vi "Get Provided Interface and Service Class.vi"(8 "error in":errorcluster, 11 "instrument in":refnum<class "ISession Factory.lvclass">) -> (0 "error out":errorcluster, 1 "service class":string, 2 "provided interface":string, 3 "instrument out":refnum<class "ISession Factory.lvclass">, 5 "using device service":bool)   [LabVIEW 2020, in "MeasurementLink Session Management V1.lvlib" / "Session Reservation.lvclass"]
uses:
  Session Reservation.lvclass
  MeasurementLink Instrument/ISession Factory/ISession Factory.lvclass
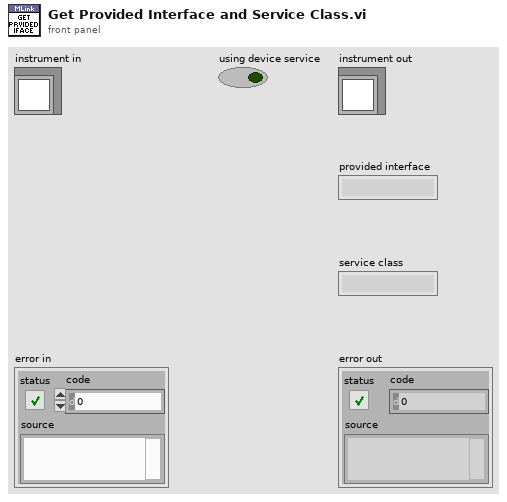
[diagram p1: front panel]
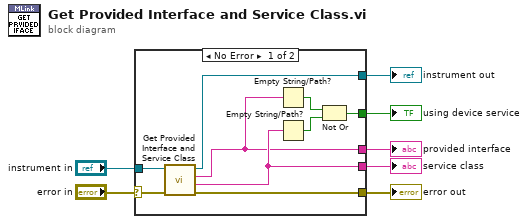
[diagram p0: block diagram]
diagram:
  n1 = case shown="No Error" "error in" {
    selector: "error in" -> [w14 w18]
    tunnel: [w16 _] -> w7
    tunnel: [w8 _] -> w6
    tunnel: [w15 _] -> w5
    tunnel: "instrument in" -> [w13 w17]
    tunnel: [w12 w18] -> w2
    tunnel: [w11 w17] -> w1
    frame No Error {
      n2 = call-dynamic "Get Provided Interface and Service Class.vi"("error in (no error)"=w14, "session factory in"=w13) -> ("error out"=w12:errorcluster, "service class"=w16:string, "provided interface"=w15:string, "session factory out"=w11:refnum<class "ISession Factory.lvclass">)  [unwired: 6 in]
      n3 = Empty String/Path?(string/path=w15) -> (empty?=w10:bool)
      n4 = Empty String/Path?(string/path=w16) -> (empty?=w9:bool)
      n5 = Not Or(1:w9, 2:w10) -> (0:w8:bool)
    }
    frame Error {
    }
  }
  "service class" <- w7
  "using device service" <- w6
  "provided interface" <- w5
  "error out" <- w2
  "instrument out" <- w1
